vi "sub_ofdm_simple_delayed_mult_CFO_sync_single.vi"(8 "CP length":i32=64, 9 "FFT size":i32=256, 11 "time samples":cdb[](array[numeric])) -> (3 "sync ofdm symbol":cdb[](array[numeric]))   [LabVIEW 2014]
panel:
  out "size(s)":i32
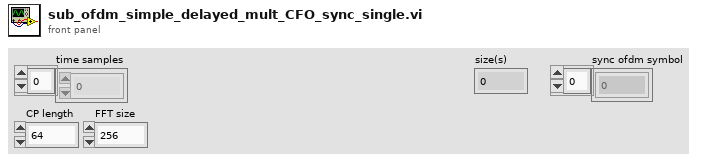
[diagram p1: front panel]
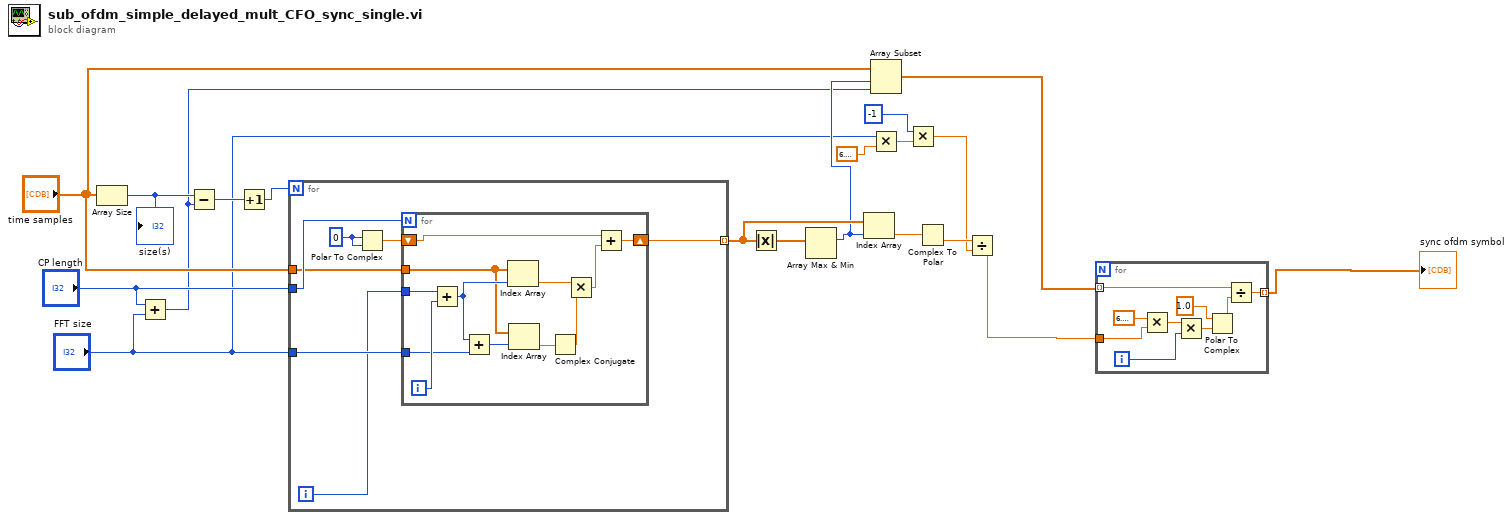
[diagram p0: block diagram]
diagram:
  n1 = Array Size(array="time samples") -> (size(s)=w7:i32)
  "size(s)" <- w7
  n2 = Add(x="CP length", y="FFT size") -> (x+y=w4:i32)
  n3 = Subtract(x=w7, y=w4) -> (x-y=w9:i32)
  n4 = Increment(x=w9) -> (x+1=w10:i32)
  n5 = for {
    N: w10 -> [_]
    tunnel: "FFT size" -> [w25]
    tunnel: "CP length" -> [w26]
    tunnel: "time samples" -> [w23]
    tunnel: [w20] -> w18 mode=indexing
    i -> [w24]
    w22 = 0
    n6 = Polar To Complex(1:w22, 2:w22) -> (0:w21:cdb)
    n7 = for {
      N: w26 -> [_]
      tunnel: w25 -> [w36]
      tunnel: w24 -> [w38]
      tunnel: w23 -> [w34]
      shift-right: [w29] -> w20
      shift-left: w21 -> [w28]
      i -> [w37]
      n8 = Add(x=w38, y=w37) -> (x+y=w35:i32)
      n9 = Add(x=w35, y=w36) -> (x+y=w33:i32)
      n10 = Index Array(array=w34, index=w35) -> (element=w31:cdb)
      n11 = Index Array(array=w34, index=w33) -> (element=w32:cdb)
      n12 = Complex Conjugate(1:w32) -> (0:w30:cdb)
      n13 = Multiply(x=w31, y=w30) -> (x*y=w27:cdb)
      n14 = Add(x=w28, y=w27) -> (x+y=w29:cdb)
    }
  }
  n15 = Absolute Value(x=w18) -> (abs(x)=w19:dbl[])
  n16 = Array Max & Min(array=w19) -> (max index (indices)=w11:i32)  [unwired: 3 out]
  n17 = Index Array(array=w18, index=w11) -> (element=w17:cdb)
  n18 = Array Subset(array="time samples", index=w11, length=w4) -> (w1:cdb[])
  n19 = Multiply(x="FFT size", y=6.283185307179586) -> (x*y=w15:dbl)
  n20 = Multiply(x=-1, y=w15) -> (x*y=w12:dbl)
  n21 = Complex To Polar(r * e^(i*theta)=w17) -> (theta=w13:dbl)  [unwired: 1 out]
  n22 = Divide(x=w13, y=w12) -> (x/y=w2:dbl)
  n23 = for {
    tunnel: w1 -> [w40] mode=indexing
    tunnel: w2 -> [w46]
    tunnel: [w39] -> w3 mode=indexing
    i -> [w44]
    n24 = Multiply(x=6.283185307179586, y=w46) -> (x*y=w45:dbl)
    n25 = Multiply(x=w45, y=w44) -> (x*y=w43:dbl)
    n26 = Polar To Complex(1:w43, 2:1.0) -> (0:w41:cdb)
    n27 = Divide(x=w40, y=w41) -> (x/y=w39:cdb)
  }
  "sync ofdm symbol" <- w3
